vi "CR-导丝纤维毛发检测2参数读取.vi"(7 "error in (no error)":errorcluster caption="错误输入（无错误）", 10 "基路径":path) -> (0 "error out":errorcluster caption="错误输出", 1 "导丝纤维毛发检测2参数":T2={"Max Number"=11.0, "Curve Extraction Settings "={"Extraction Mode"=0, "Edge Threshold"=25, "Edge Filter Size"=1, "Min Length"=19, "Row Search Step Size"=5, "Col Search Step Size"=5, "Max Endpoint Gap"=10, "Closed"=FALSE, "Subpixel"=FALSE}, "Color Mode (Histogram 1)"=0, "Range (Threshold 1)"={"Lower value"=62.0, "Upper value"=255.0}, "Clamp Settings (Max Clamp 1)"={"Angle Range (+/-)"=10.0, "Edge Polarity"={"Start"=0, "End"=0}}} {"Clamp Settings (Max Clamp 1)"."Edge Polarity"."Start" items=["Any", "Rising", "Falling"]; "Clamp Settings (Max Clamp 1)"."Edge Polarity"."End" items=["Any", "Rising", "Falling"]; "Color Mode (Histogram 1)" items=["RGB", "HSL", "HSV", "HSI"]; "Curve Extraction Settings"."Extraction Mode" items=["Normal", "Uniform Regions"]; "Curve Extraction Settings"."Edge Filter Size" items=["Fine", "Normal", "Contour Tracing"]; "Curve Extraction Settings"."Max Endpoint Gap" min=0; "Curve Extraction Settings"."Col Search Step Size" min=1 max=255 step=1; "Curve Extraction Settings"."Row Search Step Size" min=1 max=255 step=1; "Curve Extraction Settings"."Min Length" min=0; "Curve Extraction Settings"."Edge Threshold" min=1 max=350 step=1}, 2 "导丝纤维毛发检测2基础参数":T3={"IsNorImage"=TRUE, "Exposure Values"=100289, "ImagePath"=path "C:/Users/hedongpo/Desktop/514-hdp/Alignment Assemble System/Test Picture/B/3.bmp"} caption="参数界面" {"Exposure Values" scale=0.0..200000.0})   [LabVIEW 2017]
uses:
  <vilib>/vision/Pattern Matching.llb/IMAQ Curve Parameters.ctl
  <vilib>/Utility/xml.llb/Read From XML File(string).vi
  Global System.vi
panel:
  # "UI电源线反面标签1基础参数"
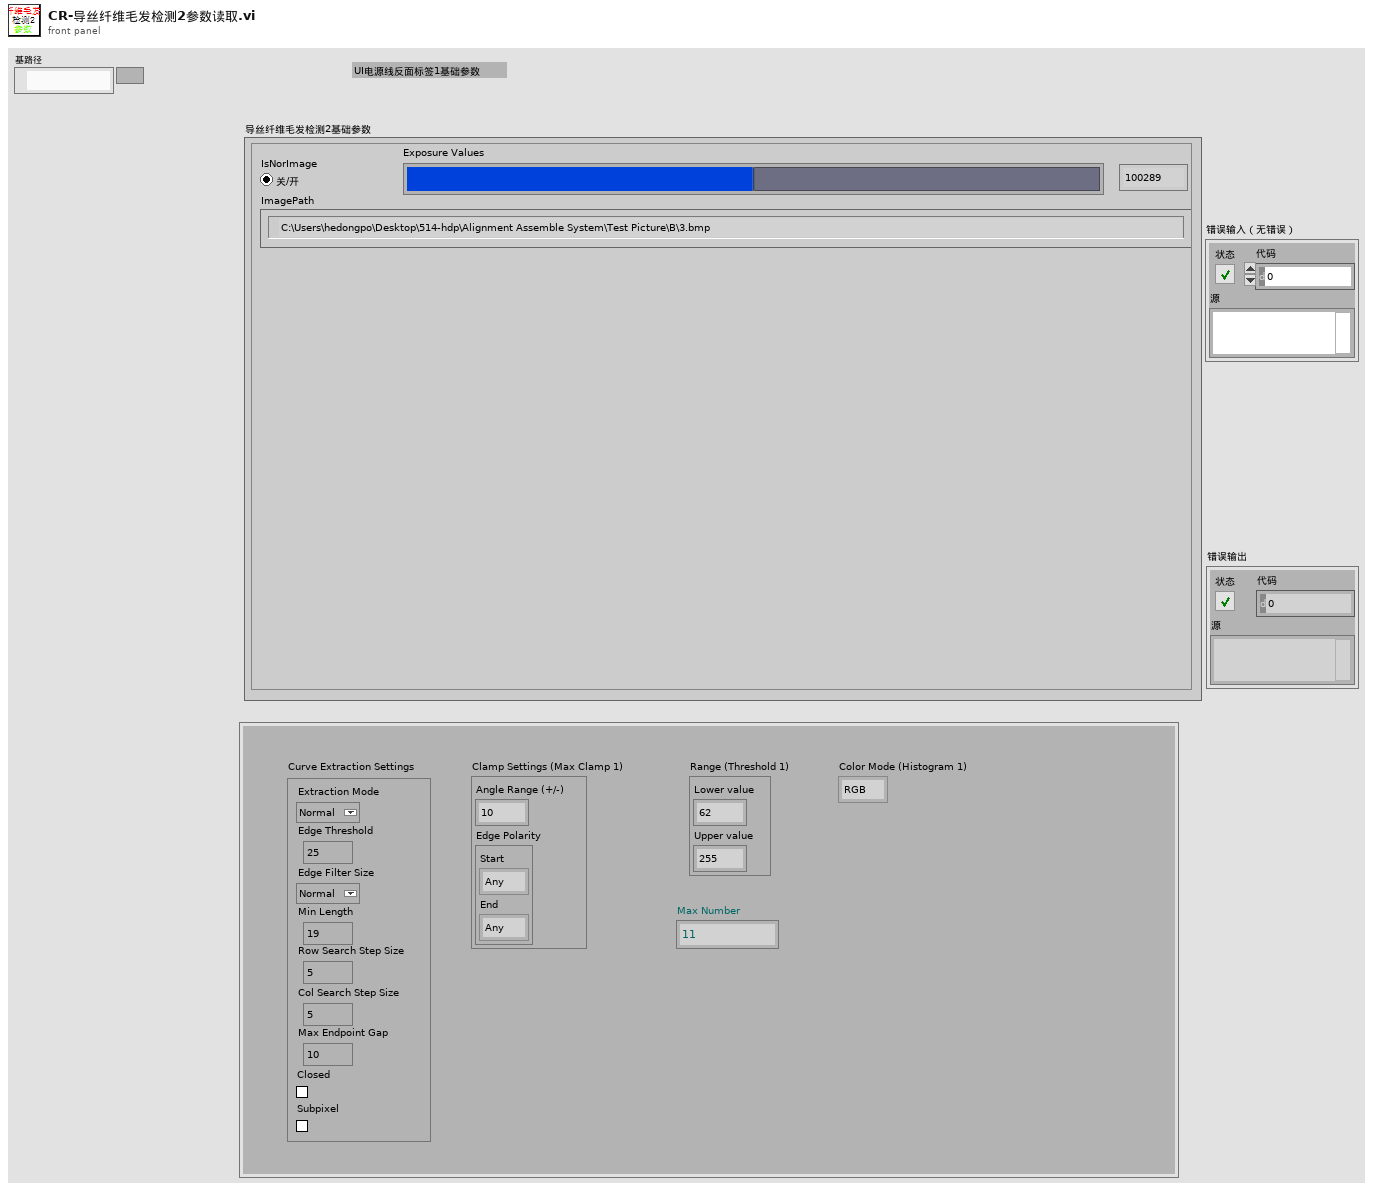
[diagram p1: front panel]
types:
  T1 = typedef "IMAQ Curve Parameters.ctl" = cluster{"Extraction Mode":u32, "Edge Threshold":i32, "Edge Filter Size":u32, "Min Length":i32, "Row Search Step Size":i32, "Col Search Step Size":i32, "Max Endpoint Gap":i32, "Closed":bool, "Subpixel":bool}
  T2 = cluster{"Max Number":sgl, "Curve Extraction Settings ":T1, "Color Mode (Histogram 1)":u16, "Range (Threshold 1)":cluster{"Lower value":sgl, "Upper value":sgl}, "Clamp Settings (Max Clamp 1)":cluster{"Angle Range (+/-)":dbl, "Edge Polarity":cluster{"Start":u32, "End":u32}}}
  T3 = cluster{"IsNorImage":bool, "Exposure Values":u32, "ImagePath":path}
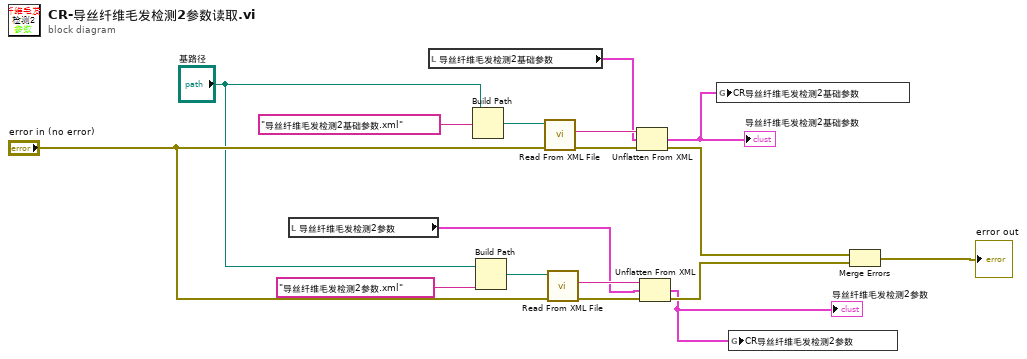
[diagram p0: block diagram]
diagram:
  n1 = local read "导丝纤维毛发检测2参数"() -> (w3:T2)
  n2 = local read "导丝纤维毛发检测2基础参数"() -> (w15:T3)
  n3 = Build Path(base path="基路径", name or relative path="导丝纤维毛发检测2基础参数.xml" ("名称或相对路径")) -> (appended path=w17:path)
  n4 = Build Path(base path="基路径", name or relative path="导丝纤维毛发检测2参数.xml" ("名称或相对路径")) -> (appended path=w6:path)
  n5 = call-poly <vilib>:"Read From XML File.vi"("error in (no error)"="error in (no error)", "XML File Path"=w17) -> ("error out"=w13:errorcluster, "XML Elements"=w16:string)  [unwired: 7 in, 1 out]
  n6 = call-poly <vilib>:"Read From XML File.vi"("error in (no error)"="error in (no error)", "XML File Path"=w6) -> ("error out"=w5:errorcluster, "XML Elements"=w7:string)  [unwired: 7 in, 1 out]
  n7 = Unflatten From XML(xml string=w16, type=w15, error in (no error)=w13) -> (value=w8:T3, error out=w12:errorcluster)
  "导丝纤维毛发检测2基础参数" <- w8
  n8 = Unflatten From XML(xml string=w7, type=w3, error in (no error)=w5) -> (value=w1:T2, error out=w4:errorcluster)
  "导丝纤维毛发检测2参数" <- w1
  n9 = global write "Global System.vi" "CR导丝纤维毛发检测2基础参数"(w8) -> ()
  n10 = global write "Global System.vi" "CR导丝纤维毛发检测2参数"(w1) -> ()
  n11 = Merge Errors(w12, w4) -> (→"error out":errorcluster)
